vi "ReadChannelStatusFpgaWithTach.vi"(7 "IEPE settling blocks":i32=20, 8 "error in":errorcluster, 10 "wfm data":waveform(sgl)[](array[waveform]), 11 "dynamic FPGA VI reference":T1) -> (0 "error out":errorcluster, 2 "wfm data":waveform(sgl)[](array[waveform]), 3 "dynamic FPGA VI reference":T1)   [LabVIEW 2017, in "cRIOWfmLib.lvlib"]
doc: "This VI sets the host application's data buffer size, which is critical for maximum data throughput. This buffer is responsible for receiving data coming from the FPGA DMA FIFO. For the continuous case the buffer size should be many times larger than your read size. In the finite case, the timing VIs automatically call this VI and set the buffer size equal to the number of samples in the acquisition."
uses:
  <vilib>/addons/InsightCM/Devices/Shared/Cms/cRIOWfmAcq/cRIOWfmLib.lvlib
  <vilib>/addons/InsightCM/Devices/Shared/Cms/cRIOWfmAcq/subVIs/RIO Wfm Cust Ctrls/rwfm_DynamicFPGAref2.ctl
  <vilib>/addons/InsightCM/Devices/Shared/Cms/cRIOWfmAcq/subVIs/stretchState.ctl
  <vilib>/Utility/error.llb/Error Cluster From Error Code.vi
  <vilib>/rvi/errors/niLvFpgaAdjustHostInterfaceError.vi
  <vilib>/rvi/interface/nirviReadWriteControl/nirviReadWriteControl.xnode
  <vilib>/addons/InsightCM/Utilities/ChannelStatus/ChannelStatus.lvlib
  NiFpgaLv.dll
  <vilib>/rvi/interface/Simulation/niFpgaSimulationCallBeginRW.vi
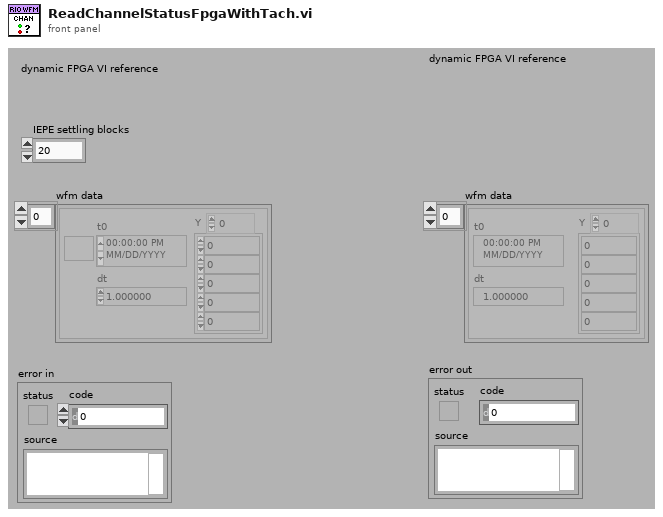
[diagram p1: front panel]
types:
  T1 = typedef "cRIOWfmLib.lvlib/rwfm_DynamicFPGAref2.ctl" = refnum<k20>
  T2 = typedef "cRIOWfmLib.lvlib/stretchState.ctl" = cluster{"input":bool, "output":bool, "pulse count":i32}
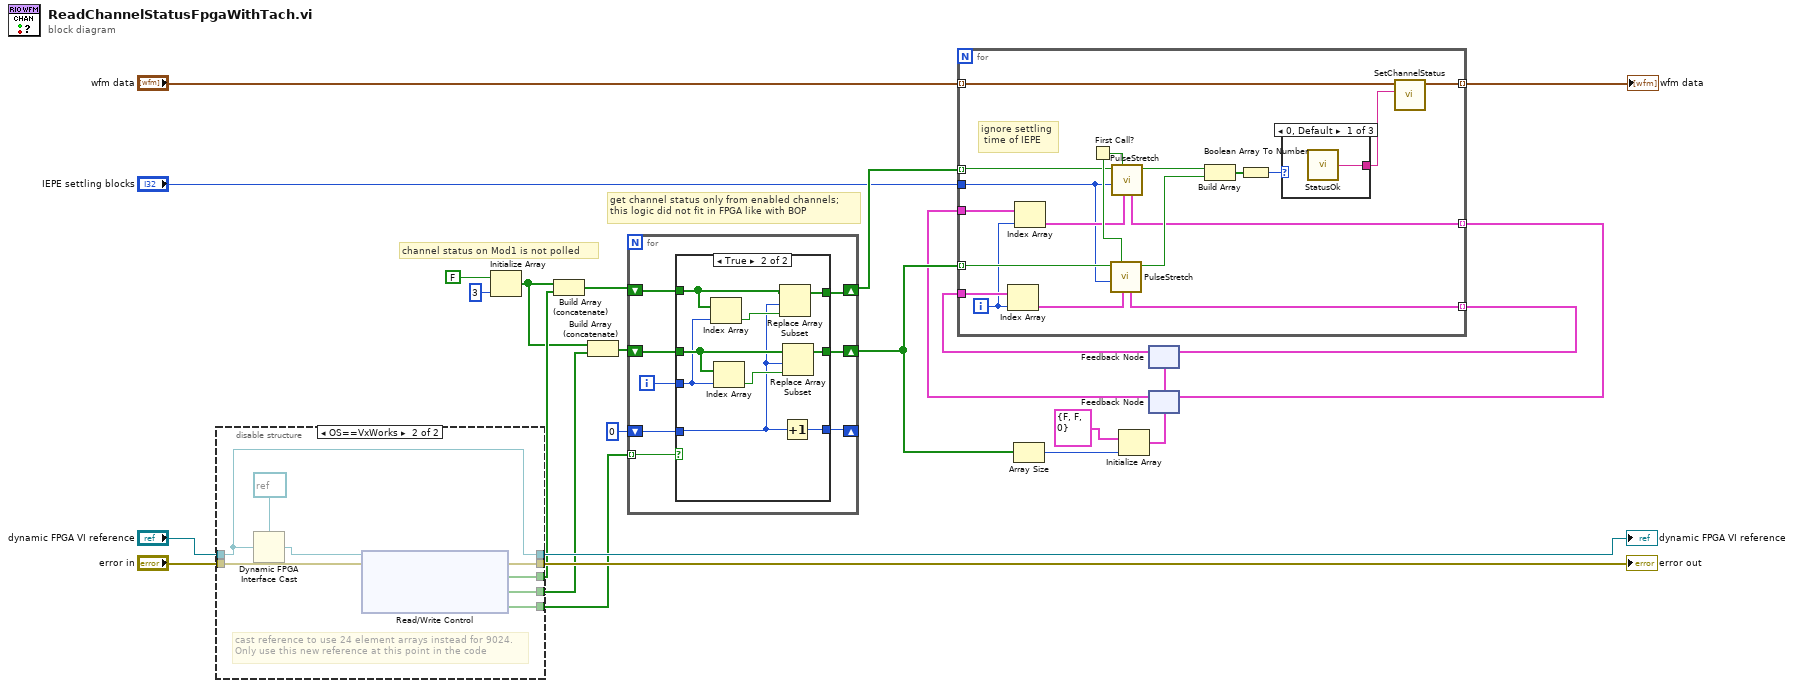
[diagram p0: block diagram]
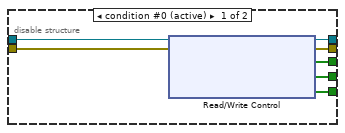
[diagram p2: hidden frame]
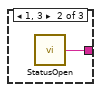
[diagram p4: hidden frame]
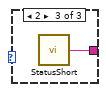
[diagram p5: hidden frame]
diagram:
  # "channel status on Mod1 is not polled"
  # "get channel status only from enabled channels;\nthis logic did not fit in FPGA like with BOP"
  n1 = disable-structure shown="OS==VxWorks" {
    disable-tunnel: "dynamic FPGA VI reference" -> [w32 w35]
    disable-tunnel: "error in" -> [w31 w40]
    disable-tunnel: [w30 w35] -> w23
    disable-tunnel: [w29 w39] -> w22
    disable-tunnel: [w28 w38] -> w19
    disable-tunnel: [w27 w37] -> w5
    disable-tunnel: [w26 w36] -> w4
    frame condition #0 (active) {
      n2 = xnode "Read/Write Control"("FPGA VI Reference In"=w32, "error in"=w31) -> ("FPGA VI Reference Out"=w30:T1, "error out"=w29:errorcluster, "Open Loop Chan Array"=w27:bool[], "Short Circuit Chan Array"=w26:bool[], "Enable Chan Array"=w28:bool[])
    }
    frame condition #1 {
      # "cast reference to use 24 element arrays instead for 9024.\nOnly use this new reference at this point in the code"
      n3 = Dynamic FPGA Interface Cast(Session In=refnum<k20> refnum ("FPGA Interface"), Type=w35) -> (Session Out=w33:refnum<k20>)
      n4 = xnode "Read/Write Control"("FPGA VI Reference In"=w33, "error in"=w40) -> ("error out"=w39:errorcluster, "Open Loop Chan Array"=w37:bool[], "Short Circuit Chan Array"=w36:bool[], "Enable Chan Array"=w38:bool[])  [unwired: 1 out]
    }
  }
  "error out" <- w22
  "dynamic FPGA VI reference" <- w23
  n5 = Initialize Array(FALSE, 3 ("dimension size")) -> (w2:bool[])
  n6 = Build Array (concatenate)(w2, w5) -> (w6:bool[])
  n7 = Build Array (concatenate)(w2, w4) -> (w3:bool[])
  n8 = for {
    tunnel: w19 -> [w48] mode=indexing
    shift-right: [w46] -> w18
    shift-left: w6 -> [w47]
    shift-right: [w43] -> _
    shift-left: 0 -> [w45]
    shift-right: [w41] -> w13
    shift-left: w3 -> [w42]
    i -> [w44]
    n9 = case shown="True" w48 {
      tunnel: w47 -> [w51 w59]
      tunnel: [w51 w58] -> w46
      tunnel: w45 -> [w50 w54]
      tunnel: w44 -> [_ w53]
      tunnel: [w50 w57] -> w43
      tunnel: w42 -> [w49 w55]
      tunnel: [w49 w52] -> w41
      frame False {
      }
      frame True {
        n10 = Index Array(array=w59, index=w53) -> (element=w60:bool)
        n11 = Index Array(array=w55, index=w53) -> (element=w56:bool)
        n12 = Replace Array Subset(array=w59, new element=w60, index=w54) -> (w58:bool[])
        n13 = Increment(x=w54) -> (x+1=w57:i32)
        n14 = Replace Array Subset(array=w55, new element=w56, index=w54) -> (w52:bool[])
      }
    }
  }
  n15 = Array Size(array=w13) -> (size(s)=w16:i32)
  n16 = Initialize Array(T2 {"input"=FALSE, "output"=FALSE, "pulse count"=0} ("element"), w16) -> (w14:T2[])
  n17 = feedback #1(w14) -> (w11:T2[])
  n18 = feedback #2(w14) -> (w9:T2[])
  n19 = for {
    tunnel: "wfm data" -> [w64] mode=indexing
    tunnel: w18 -> [w77] mode=indexing
    tunnel: w13 -> [w76] mode=indexing
    tunnel: [w63] -> w20 mode=indexing
    tunnel: [w73] -> w12 mode=indexing
    tunnel: w11 -> [w72]
    tunnel: [w69] -> w10 mode=indexing
    tunnel: w9 -> [w68]
    tunnel: "IEPE settling blocks" -> [w66]
    i -> [w70]
    # "ignore settling\n time of IEPE"
    n20 = Index Array(array=w72, index=w70) -> (element=w71:T2)
    n21 = Index Array(array=w68, index=w70) -> (element=w67:T2)
    n22 = First Call?() -> (First Call?: T/F=w78:bool)
    n23 = call <vilib>:"PulseStretch.vi"("state in"=w71, "Reset"=w78, "Pulse Width"=w66, "Input"=w76) -> ("Output"=w74:bool, "state out"=w73:T2)  [unwired: 6 in]
    n24 = call <vilib>:"PulseStretch.vi"("state in"=w67, "Reset"=w78, "Pulse Width"=w66, "Input"=w77) -> ("Output"=w75:bool, "state out"=w69:T2)  [unwired: 6 in]
    n25 = Build Array(w75, w74) -> (w62:bool[])
    n26 = Boolean Array To Number(Boolean array=w62) -> (number=w61:u32)
    n27 = case shown="0, Default" w61 {
      tunnel: [w79 w80 w81] -> w65
      frame 0, Default {
        n28 = call <vilib>:"StatusOk.vi"() -> ("status"=w79:string)  [unwired: 5 in]
      }
      frame 1, 3 {
        n29 = call <vilib>:"StatusOpen.vi"() -> ("status"=w80:string)  [unwired: 5 in]
      }
      frame 2 {
        n30 = call <vilib>:"StatusShort.vi"() -> ("status"=w81:string)  [unwired: 5 in]
      }
    }
    n31 = call <vilib>:"SetChannelStatus.vi"("Channel Status"=w65, "Waveform in"=w64) -> ("Waveform out"=w63:waveform(sgl))  [unwired: 8 in, 1 out]
  }
  "wfm data" <- w20
  n32 = feedback-in #1(w12) -> ()
  n33 = feedback-in #2(w10) -> ()
